vi "字符串映射表.vi"(0 "输入字符串":string, 1 "映射表":u8[](array[numeric])) -> (2 "输出字符串":string)   [LabVIEW 2012]
doc: "Maps characters in \"text in\" according to \"map\".\n\nIf \"map\" is an array of 256 elements, then\n\n text_out[i] = map[ text_in[i] ]\n\notherwise\n\n text_out[i] = text_i [i]"
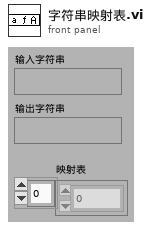
[diagram p1: front panel]
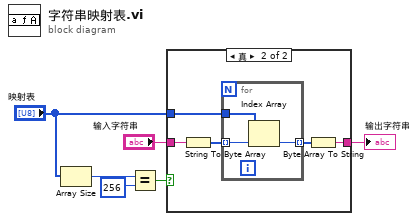
[diagram p0: block diagram]
diagram:
  n1 = Array Size(array="映射表") -> (size(s)=w4:i32)
  n2 = Equal?(x=w4, y=256) -> (x = y?=w2:bool)
  n3 = case shown="真" w2 {
    tunnel: [w7 w12] -> w5
    tunnel: "输入字符串" -> [w7 w10]
    tunnel: "映射表" -> [_ w9]
    frame False {
    }
    frame True {
      n4 = String To Byte Array(string=w10) -> (unsigned byte array=w11:u8[])
      n5 = for {
        tunnel: w11 -> [w15] mode=indexing
        tunnel: w9 -> [w13]
        tunnel: [w14] -> w8 mode=indexing
        n6 = Index Array(array=w13, index=w15) -> (element=w14:u8)
      }
      n7 = Byte Array To String(unsigned byte array=w8) -> (string=w12:string)
    }
  }
  "输出字符串" <- w5
